vi "AlphaBetaToDQ_noSine_src.vi"(0 "alpha":sgl format="%#_32g", 1 "cosx":sgl, 2 "sinx":sgl, 5 "beta":sgl format="%#_32g") -> (4 "direct":sgl, 6 "quadrature":sgl)   [LabVIEW 2015]
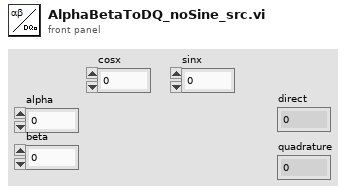
[diagram p1: front panel]
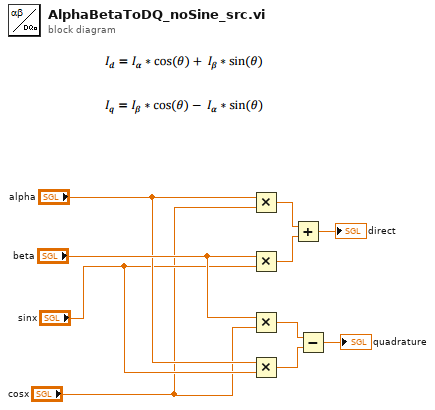
[diagram p0: block diagram]
diagram:
  n1 = Multiply(x="alpha", y="cosx") -> (x*y=w8:sgl)
  n2 = Multiply(x="beta", y="sinx") -> (x*y=w7:sgl)
  n3 = Multiply(x="beta", y="cosx") -> (x*y=w6:sgl)
  n4 = Multiply(x="alpha", y="sinx") -> (x*y=w5:sgl)
  n5 = Add(x=w8, y=w7) -> (x+y=→"direct":sgl)
  n6 = Subtract(x=w6, y=w5) -> (x-y=→"quadrature":sgl)
